vi "Gasteiler initialisieren.vi"(11 "Gasteiler Referenz":refnum<vi>) -> ()   [LabVIEW 2020, in "System Einstellungen V2.lvlib"]
uses:
  System Einstellungen V2.lvlib
  <vilib>/Utility/miscctls.llb/LVStringsAndValuesArrayTypeDef.ctl
  Aktion FGV SystemEinstellungenV2.ctl
panel:
  in  "Strings und Werte []":T1
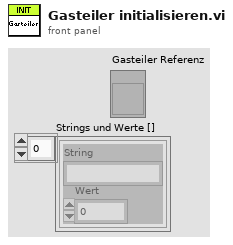
[diagram p1: front panel]
types:
  T1 = typedef "LVStringsAndValuesArrayTypeDef.ctl" = cluster{"String":string, "Value":ext}[]
  T2 = typedef "System Einstellungen V2.lvlib/Aktion FGV SystemEinstellungenV2.ctl" = enum16{"lesen", "Analysatoren schreiben", "Analysator ändern", "Analysatoren löschen", "laden", "speichern", "Untertitel", "Analysatoren", "Neue Analysatoren", "Gasteiler schreiben", "Gasteiler ändern", "Gasteiler löschen", "Gasteiler", "Gasteiler exportieren", "Gasteiler importieren"}
  T3 = typedef "System Einstellungen V2.lvlib/Gasteiler.ctl" = cluster{"Gasteiler Name":string, "Gasteiler Type":string, "Gasteiler Seriennummer":string, "Gasteiler Letzte Wartung":timestamp}
  T4 = cluster{"GasteilerDefinitionsListe":T3[], "GasteilerDefinitionTextliste":string[][], "Gasteiler Strings And Values":cluster{"String":string, "Wert":string}[]}
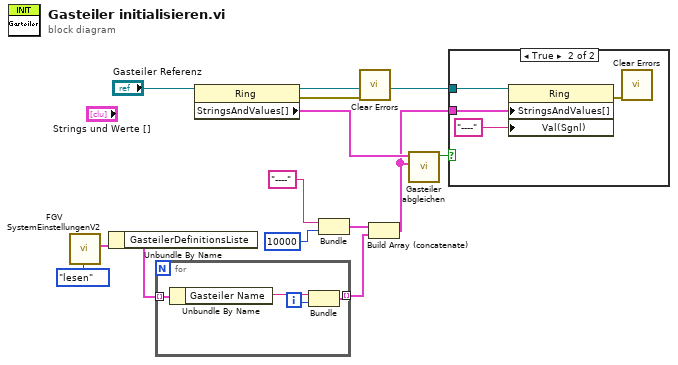
[diagram p0: block diagram]
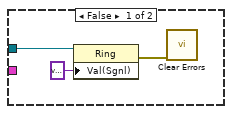
[diagram p2: hidden frame]
diagram:
  n1 = call "FGV SystemEinstellungenV2.vi"("Aktion"=Aktion_FGV_SystemEinstellungenV2."lesen") -> ("Gasteiler"=w10:T4)  [unwired: 5 in, 5 out]
  n2 = Unbundle By Name(w10) -> ("GasteilerDefinitionsListe"=w11:T3[])
  n3 = for {
    tunnel: w11 -> [w17] mode=indexing
    tunnel: [w14] -> w2 mode=indexing
    i -> [w15]
    n4 = Unbundle By Name(w17) -> ("Gasteiler Name"=w16:string)
    n5 = Bundle("Gasteiler Name"=w16, w15) -> (w14:cluster{"Gasteiler Name":string, i32})  [unwired: 1 in]
  }
  n6 = property on="Eigenschaftsknoten" class="Ring"(reference="Gasteiler Referenz") -> (reference out=w7:refnum<vi>, error out=w8:errorcluster, "StringsAndValues[]"=w9:T1)  [unwired: 1 in]
  n7 = Bundle("----", 10000) -> (w3:cluster{string, i32})  [unwired: 1 in]
  n8 = call <vilib>:"Clear Errors.vi"("error in (no error)"=w8) -> ()  [unwired: 5 in, 2 out]
  n9 = Build Array (concatenate)(w3, w2) -> (w1:cluster{"Gasteiler Name":string, i32}[])
  n10 = call "Gasteiler abgleichen.vi"("Gasteiler"=w1, "Gasteilerliste"=w9) -> ("x != y?"=w13:bool)  [unwired: 9 in]
  n11 = case shown="True" w13 {
    tunnel: w7 -> [w18 w22]
    tunnel: w1 -> [_ w23]
    frame False {
      n12 = property class="Ring"(reference=w18, "Val(Sgnl)"=variant ("Wert (signalisierend)")) -> (error out=w20:errorcluster)  [unwired: 1 in, 1 out]
      n13 = call <vilib>:"Clear Errors.vi"("error in (no error)"=w20) -> ()  [unwired: 5 in, 2 out]
    }
    frame True {
      n14 = property class="Ring"(reference=w22, "StringsAndValues[]"=w23, "Val(Sgnl)"="----" ("Value")) -> (error out=w24:errorcluster)  [unwired: 1 in, 1 out]
      n15 = call <vilib>:"Clear Errors.vi"("error in (no error)"=w24) -> ()  [unwired: 5 in, 2 out]
    }
  }
